vi "Config Folder.vi"() -> (3 ".config folder":path)   [LabVIEW 2019, in "SLMP.lvlib"]
uses:
  SLMP.lvlib
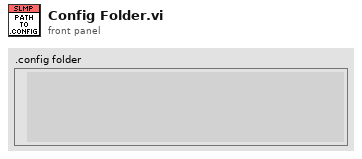
[diagram p1: front panel]
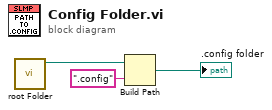
[diagram p0: block diagram]
diagram:
  n1 = call "root Folder.vi"() -> ("root folder"=w2:path)  [unwired: 11 in]
  n2 = Build Path(base path=w2, name or relative path=".config") -> (appended path=→".config folder":path)
